vi "Facade.vi"(0 "Data In":T10, 2 "Display State In":T5={"ImageSource"=enum."Camera", "IMAQdx Cam"=refnum, "WorkDir"=path "", "Image Name Prefix"="", "ROI"={"Global Rectangle"=[], "Contours"=[]}, "BG Image"=refnum, "Display Image"=refnum, "Display settings"={"Min. Thresh."=0.0, "X"=0.0, "Y"=0.0, "ShowLineout"=FALSE, "ScaleParts"=10, "ShowLegende"=FALSE, "Target Cross"=FALSE, "Centroid Cross"=FALSE, "Target color"=16777226, "Centroid color"=16711680, "calibr. mm/px"=0.0}, "Mask image"=refnum, "ConfigDir"=path "", "Display ref"=refnum, "Saved ROIs"=[], "Selected ROI"="", "Analyze Objects"=[], "Analysis Params"=variant, "Analysis Results"=variant, "Overlays?"=[], "Ref Palette type"=refnum, "Time in Filename?"=TRUE, "Save Report?"=TRUE, "Appl Params"=variant, "Show ZoomBtn?"=TRUE, "Image file"=path ""} {"ROI"."Contours"."Type" items=["No Selection", "Point", "Line", "Rectangle", "Oval", "Polygon", "Freehand Region", "Annulus", "Unused2", "Unused3", "Broken Line", "Freehand Line", "Rotated Rectangle"]}, 3 "Container State":T9) -> (6 "Data Out":T10, 7 "Display State Out":T5={"ImageSource"=enum."Camera", "IMAQdx Cam"=refnum, "WorkDir"=path "", "Image Name Prefix"="", "ROI"={"Global Rectangle"=[], "Contours"=[]}, "BG Image"=refnum, "Display Image"=refnum, "Display settings"={"Min. Thresh."=0.0, "X"=0.0, "Y"=0.0, "ShowLineout"=FALSE, "ScaleParts"=10, "ShowLegende"=FALSE, "Target Cross"=FALSE, "Centroid Cross"=FALSE, "Target color"=16777226, "Centroid color"=16711680, "calibr. mm/px"=0.0}, "Mask image"=refnum, "ConfigDir"=path "", "Display ref"=refnum, "Saved ROIs"=[], "Selected ROI"="", "Analyze Objects"=[], "Analysis Params"=variant, "Analysis Results"=variant, "Overlays?"=[], "Ref Palette type"=refnum, "Time in Filename?"=TRUE, "Save Report?"=TRUE, "Appl Params"=variant, "Show ZoomBtn?"=TRUE, "Image file"=path ""} {"ROI"."Contours"."Type" items=["No Selection", "Point", "Line", "Rectangle", "Oval", "Polygon", "Freehand Region", "Annulus", "Unused2", "Unused3", "Broken Line", "Freehand Line", "Rotated Rectangle"]}, 8 "Action":T4)   [LabVIEW 2020, in "POLARIS IMAQ Display.xctl"]
uses:
  POLARIS IMAQ Display.xctl
  Data.ctl
  <vilib>/vision/Image Controls.llb/IMAQ Image.ctl
  <vilib>/_xctls/Container State.ctl
  State.ctl
  IMAQdx Cam/IMAQdx Cam.lvclass
  Properties/ImageSource.ctl
  DisplaySettings.ctl
  Named ROI.ctl
  Analyze Classes/Analyze BaseClass/Analyze BaseClass.lvclass
  Palette.ctl
  <vilib>/_xctls/Action.ctl
  <vilib>/_xctls/XControlSupport.lvlib
  Utility/POLARIS Vision utility.lvlib
  <vilib>/vision/NI_Vision_Development_Module.lvlib
  <vilib>/Utility/config.llb/NI_LVConfig.lvlib
panel:
  in  "Zoom Buttons":enum32{"Zoom in", "Zoom out", "Zenter"}(radio)
  in  "Pallete":T1={"Teiler"=1, "Palette Type"=0} {"Teiler" min=1 max=5; "Palette Type" items=["Grayscale", "Binary", "Gradient", "Rainbow", "Temperature", "User Defined"]}
  in  "Report File":path
  in  "ROI Name":string
  out "Display settings":T2={"Min. Thresh."=0.0, "X"=0.0, "Y"=0.0, "ShowLineout"=FALSE, "ScaleParts"=10, "ShowLegende"=FALSE, "Target Cross"=FALSE, "Centroid Cross"=FALSE, "Target color"=16777226, "Centroid color"=16711680, "calibr. mm/px"=0.0}
  out "Centroid":cluster{"X Centroid":sgl, "Y Centroid":sgl} {"Y Centroid" format="%.2f"; "X Centroid" format="%.2f"}
  in  "Sub\nBG":bool
  out "error out":errorcluster
  out "Image":T3(plugin-control)
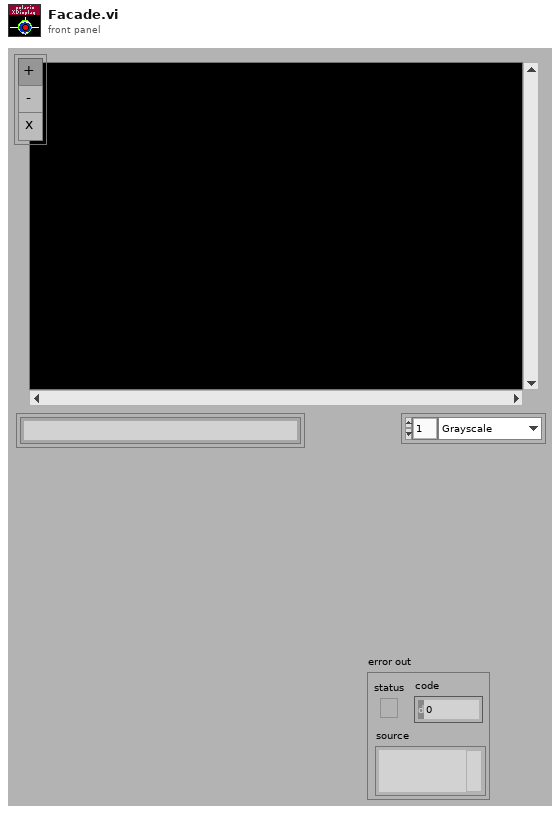
[diagram p1: front panel]
types:
  T1 = typedef "POLARIS IMAQ Display.xctl/Palette.ctl" = cluster{"Teiler":i32, "Palette Type":u32}
  T2 = typedef "POLARIS IMAQ Display.xctl/DisplaySettings.ctl" = cluster{"Min. Thresh.":sgl, "X":dbl, "Y":dbl, "ShowLineout":bool, "ScaleParts":i32, "ShowLegende":bool, "Target Cross":bool, "Centroid Cross":bool, "Target color":u32, "Centroid color":u32, "calibr. mm/px":sgl}
  T3 = typedef "IMAQ Image.ctl" = refnum<image>
  T4 = typedef "XControlSupport.lvlib/Action.ctl" = cluster{"Data Changed?":bool, "State Changed?":bool, "Action Name":string}
  T5 = typedef "POLARIS IMAQ Display.xctl/State.ctl" = cluster{"ImageSource":T6, "IMAQdx Cam":refnum<class "IMAQdx Cam.lvclass">, "WorkDir":path, "Image Name Prefix":string, "ROI":T7, "BG Image":T3, "Display Image":T3, "Display settings":T2, "Mask image":T3, "ConfigDir":path, "Display ref":refnum<vi>, "Saved ROIs":T8[], "Selected ROI":string, "Analyze Objects":refnum<class "Analyze BaseClass.lvclass">[], "Analysis Params":variant, "Analysis Results":variant, "Overlays?":bool[], "Ref Palette type":refnum<vi>, "Time in Filename?":bool, "Save Report?":bool, "Appl Params":variant, "Show ZoomBtn?":bool, "Image file":path}
  T6 = typedef "POLARIS IMAQ Display.xctl/ImageSource.ctl" = enum16{"Camera", "File"}
  T7 = typedef "ROI Descriptor" = cluster{"Global Rectangle":i32[], "Contours":cluster{"ID":enum32{"External", "Internal"}, "Type":u32, "Coordinates":i32[]}[]}
  T8 = typedef "POLARIS IMAQ Display.xctl/Named ROI.ctl" = cluster{"ROI":cluster{"Global Rectangle":i32[], "Contours":cluster{"Contour Type":u32, "ROI Type":u32, "Points":i32[]}[]}, "Name":string}
  T9 = typedef "XControlSupport.lvlib/Container State.ctl" = cluster{"Indicator?":bool, "Run Mode?":bool, " Refnum":refnum<vi>}
  T10 = typedef "POLARIS IMAQ Display.xctl/Data.ctl" = cluster{"Image":T3}
  T11 = typedef "Image Type" = u32
  T12 = cluster{"Global Rectangle":i32[], "Contours":cluster{"Contour Type":u32, "ROI Type":u32, "Points":i32[]}[]}
  T13 = typedef "IMAQdx.ctl" = refnum<k21>
  T14 = typedef "NI_LVConfig.lvlib/Config Data RefNum.ctl" = refnum<k1>
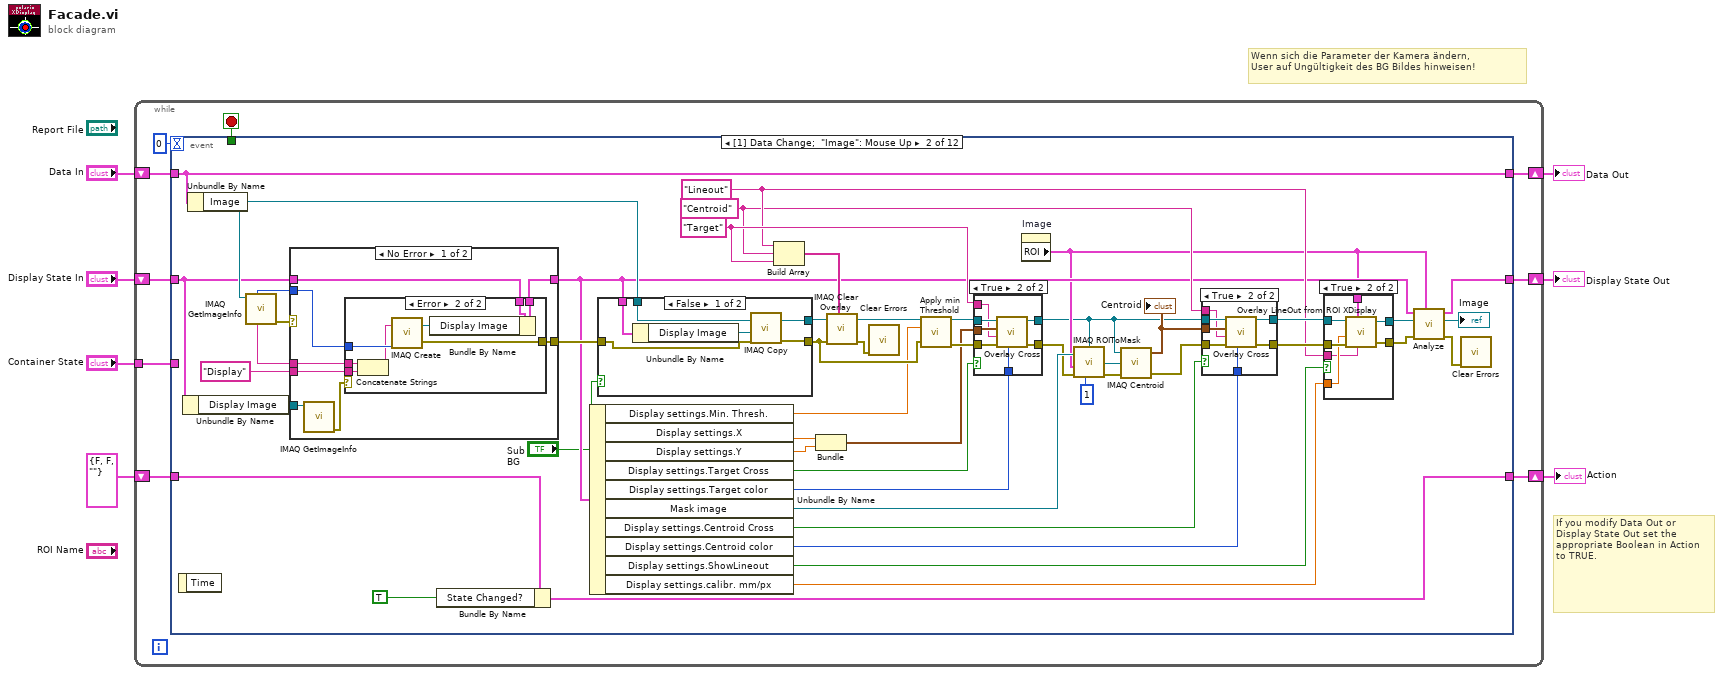
[diagram p0: block diagram]
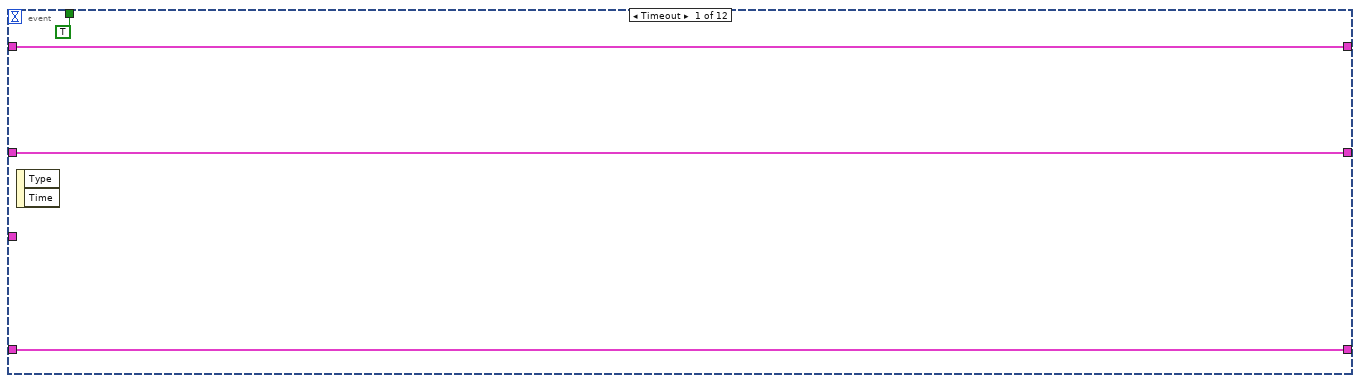
[diagram p2: hidden frame]
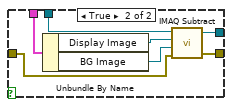
[diagram p8: hidden frame]
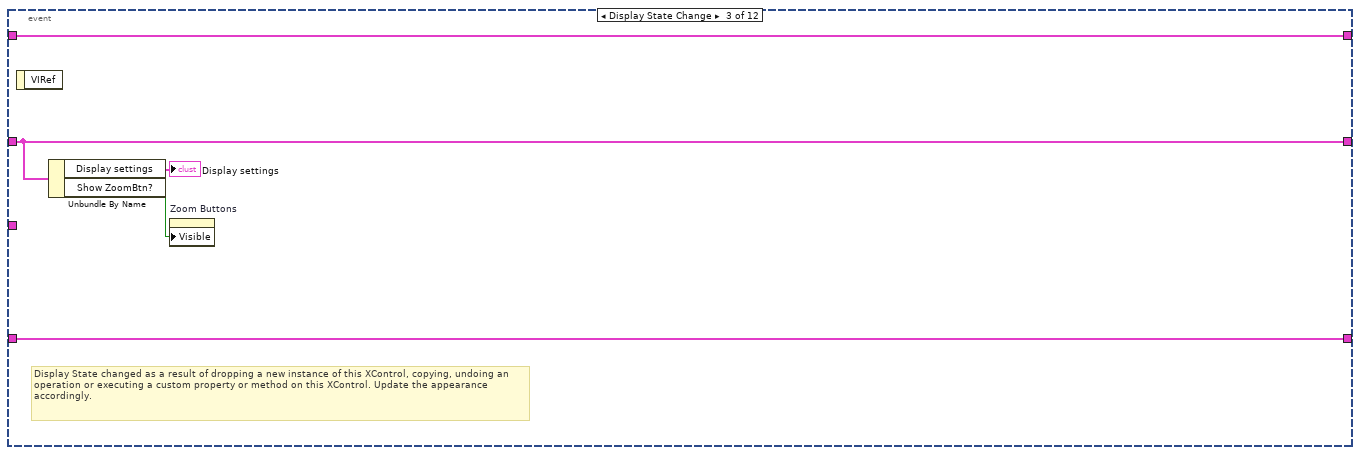
[diagram p9: hidden frame]
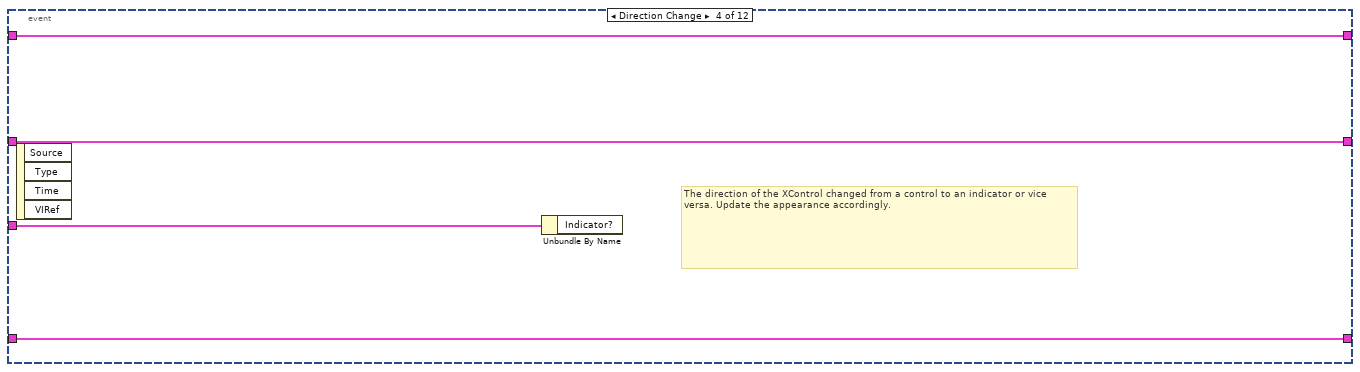
[diagram p10: hidden frame]
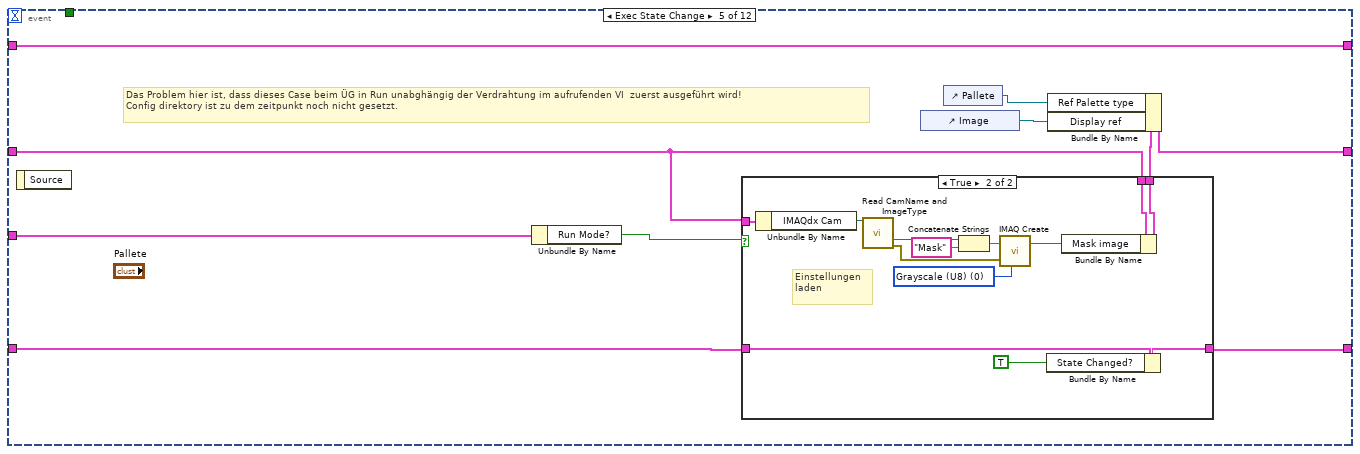
[diagram p11: hidden frame]
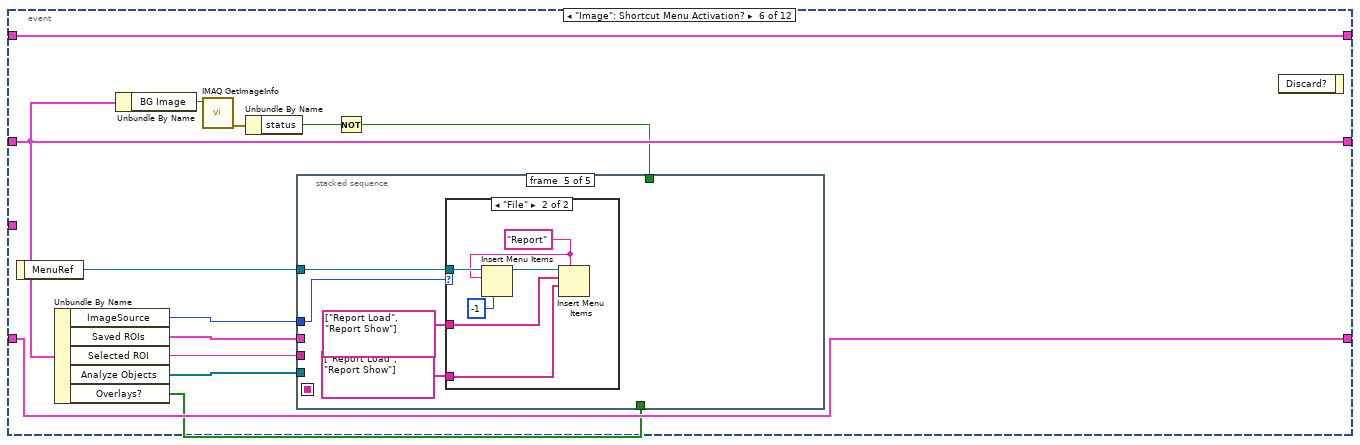
[diagram p13: hidden frame]
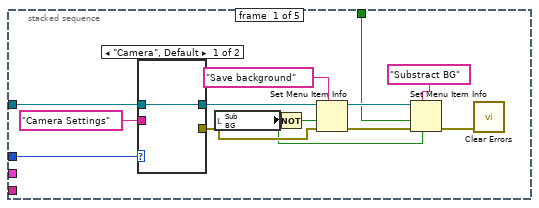
[diagram p14: hidden frame]
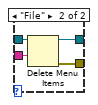
[diagram p15: hidden frame]
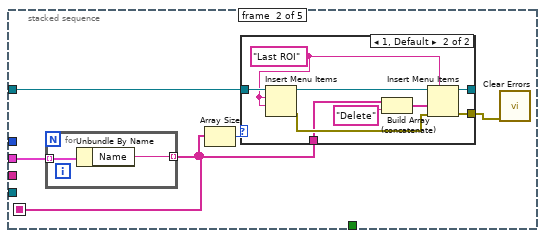
[diagram p16: hidden frame]
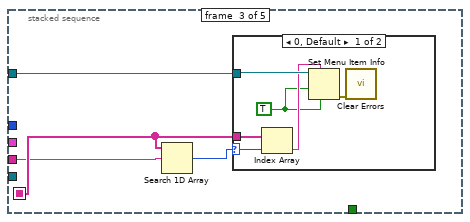
[diagram p18: hidden frame]
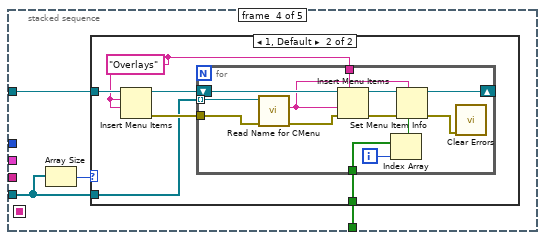
[diagram p20: hidden frame]
diagram:
  # "Wenn sich die Parameter der Kamera ändern,\nUser auf Ungültigkeit des BG Bildes hinweisen!"
  # "If you modify Data Out or\nDisplay State Out set the\nappropriate Boolean in Action\nto TRUE."
  n1 = while {
    shift-right: [w15] -> w4
    shift-left: "Display State In" -> [w16]
    tunnel: "Container State" -> [w12]
    shift-right: [w11] -> w7
    shift-left: "Data In" -> [w8]
    shift-right: [w9] -> w2
    shift-left: T4 {"Data Changed?"=FALSE, "State Changed?"=FALSE, "Action Name"=""} ("Action") -> [w10]
    stop <- w14 stop-if-true
    n2 = event shown="[1] Data Change;  \"Image\": Mouse Up" {
      selector: _ -> [_ _ _ _ _ _ _ _ _ _ _ _]
      dyn-events: _ -> [_ _ _ _ _ _ _ _ _ _ _ _]
      timeout: 0 -> [_ _ _ _ _ _ _ _ _ _ _ _]
      tunnel: w16 -> [w18 w23 w131 w137 w145 w174 w260 w426 w437 w451 w457 w462]
      tunnel: [w18 w32 w131 w137 w141 w174 w258 w425 w431 w442 w457 w462] -> w15
      tunnel: [TRUE _ _ _ _ _ _ _ _ _ _ _] -> w14
      tunnel: w12 -> [_ _ _ w138 w148 _ w255 _ _ _ _ _]
      tunnel: w8 -> [w17 w70 w134 w136 w147 w176 w259 w429 w441 w450 w456 w461]
      tunnel: [w17 w70 w134 w136 w147 w176 w259 w429 w441 w450 w456 w461] -> w11
      tunnel: [w19 w46 w132 w135 w142 w175 w256 w416 w434 w448 w455 w460] -> w9
      tunnel: w10 -> [w19 w47 w132 w135 w143 w175 w257 w428 w440 w449 w455 w460]
      event Timeout {
        n3 = event-data() -> ()  [unwired: 1 in, 2 out]
      }
      event Data Change; "Image": Mouse Up {
        w38 = "Lineout" ("Group")
        w39 = "Target"
        w37 = "Centroid"
        n4 = event-data() -> ()  [unwired: 1 in, 1 out]
        n5 = Unbundle By Name(w23) -> ("Display Image"=w22:T3)
        n6 = Unbundle By Name(w70) -> ("Image"=w44:T3)
        n7 = call "IMAQ GetImageInfo"("Image"=w44) -> ("error out"=w41:errorcluster, "Image Name"=w43:string, "Image Type"=w42:T11)  [unwired: 3 in, 5 out]
        n8 = case shown="No Error" w41 {
          selector: w41 -> [_ w88]
          tunnel: w23 -> [w78 w89]
          tunnel: [w77 w89] -> w33
          tunnel: [w76 w88] -> w45
          tunnel: w43 -> [w75 _]
          tunnel: w42 -> [w74 _]
          tunnel: "Display" ("string") -> [w73 _]
          tunnel: w22 -> [w72 _]
          frame No Error {
            n9 = call "IMAQ GetImageInfo"("Image"=w72) -> ("error out"=w71:errorcluster)  [unwired: 3 in, 7 out]
            n10 = case shown="Error" w71 {
              tunnel: w78 -> [w79 w87]
              tunnel: [w79 w86] -> w77
              tunnel: [_ w85] -> w76
              tunnel: w75 -> [_ w84]
              tunnel: w74 -> [_ w83]
              tunnel: w73 -> [_ w80]
              frame No Error {
              }
              frame Error {
                n11 = Concatenate Strings(w84, w80) -> (w82:string)
                n12 = call "IMAQ Create"("Image Name"=w82, "Image Type"=w83) -> ("New Image"=w81:T3, "error out"=w85:errorcluster)  [unwired: 3 in]
                n13 = Bundle By Name(cluster=w87, "Display Image"=w81) -> (w86:T5)
              }
            }
          }
          frame Error {
          }
        }
        n14 = Bundle By Name(cluster=w47, "State Changed?"=TRUE) -> (w46:T4)
        n15 = Unbundle By Name(w33) -> ("Display settings.Min. Thresh."=w24:sgl, "Display settings.X"=w67:dbl, "Display settings.Y"=w66:dbl, "Display settings.Target Cross"=w65:bool, "Display settings.Target color"=w63:u32, "Mask image"=w59:T3, "Display settings.Centroid Cross"=w58:bool, "Display settings.Centroid color"=w55:u32, "Display settings.ShowLineout"=w51:bool, "Display settings.calibr. mm/px"=w50:sgl)
        n16 = case shown="False" "Sub\nBG" {
          tunnel: w33 -> [w122 w129]
          tunnel: w44 -> [w121 w126]
          tunnel: [w119 w127] -> w49
          tunnel: [w118 w124] -> w35
          tunnel: w45 -> [w117 w123]
          frame False {
            n17 = Unbundle By Name(w122) -> ("Display Image"=w120:T3)
            n18 = call "IMAQ Copy"("error in (no error)"=w117, "Image Dst"=w120, "Image Src"=w121) -> ("error out"=w118:errorcluster, "Image Dst Out"=w119:T3)  [unwired: 3 in]
          }
          frame True {
            n19 = Unbundle By Name(w129) -> ("Display Image"=w125:T3, "BG Image"=w128:T3)
            n20 = call "IMAQ Subtract"("Image Src A"=w126, "Image Dst"=w125, "Image Src B"=w128, "error in (no error)"=w123) -> ("Image Dst Out"=w127:T3, "error out"=w124:errorcluster)  [unwired: 3 in]
          }
        }
        n21 = Build Array(w38, w37, w39) -> (w36:string[])
        n22 = Bundle("X"=w67, "Y"=w66) -> (w64:cluster{"X":dbl, "Y":dbl})  [unwired: 1 in]
        n23 = call "IMAQ Clear Overlay"("Groups"=w36, "error in (no error)"=w35, "Image"=w49) -> ("error out"=w34:errorcluster, "Image Out"=w48:T3)  [unwired: 7 in]
        n24 = call <vilib>:"Clear Errors.vi"("error in (no error)"=w34) -> ()  [unwired: 5 in, 2 out]
        n25 = call "Apply min Threshold.vi"("error in"=w35, "Min. Thresh."=w24, "Image In"=w48) -> ("error out"=w68:errorcluster, "Image Out"=w69:T3)  [unwired: 7 in]
        n26 = case shown="True" w65 {
          tunnel: w69 -> [w109 w116]
          tunnel: [w109 w115] -> w21
          tunnel: w68 -> [w108 w114]
          tunnel: w64 -> [_ w113]
          tunnel: w63 -> [_ w112]
          tunnel: [w108 w111] -> w57
          tunnel: w39 -> [_ w110]
          frame False {
          }
          frame True {
            n27 = call "Overlay Cross.vi"("Color"=w112, "error in (no error)"=w114, "Overlay Group"=w110, "point"=w113, "Image In"=w116) -> ("error out"=w111:errorcluster, "Image Out"=w115:T3)  [unwired: 4 in]
          }
        }
        n28 = property on="Image" class="ImageControl"() -> ("ROI"=w27:T12)  [unwired: 2 in, 2 out]
        n29 = call "IMAQ ROIToMask"("error in (no error)"=w57, "ROI Descriptor"=w27, "Filling Value (255)"=1, "Image"=w59, "Image Model"=w21) -> ("error out"=w62:errorcluster, "Image Out"=w61:T3)  [unwired: 1 in, 1 out]
        n30 = call "IMAQ Centroid"("error in (no error)"=w62, "Image Mask"=w61, "Image"=w21) -> ("error out"=w56:errorcluster, "Centroid"=w54:cluster{"X Centroid":sgl, "Y Centroid":sgl})  [unwired: 1 in]
        "Centroid" <- w54
        n31 = case shown="True" w58 {
          tunnel: w21 -> [w100 w107]
          tunnel: [w100 w106] -> w53
          tunnel: w56 -> [w99 w105]
          tunnel: w54 -> [_ w104]
          tunnel: w55 -> [_ w103]
          tunnel: [w99 w102] -> w52
          tunnel: w37 -> [_ w101]
          frame False {
          }
          frame True {
            n32 = call "Overlay Cross.vi"("Color"=w103, "error in (no error)"=w105, "Overlay Group"=w101, "point"=w104, "Image In"=w107) -> ("error out"=w102:errorcluster, "Image Out"=w106:T3)  [unwired: 4 in]
          }
        }
        n33 = case shown="True" w51 {
          tunnel: w53 -> [w91 w98]
          tunnel: w52 -> [w90 w97]
          tunnel: w27 -> [_ w96]
          tunnel: [w91 w95] -> w31
          tunnel: [w90 w94] -> w29
          tunnel: w50 -> [_ w93]
          tunnel: w38 -> [_ w92]
          frame False {
          }
          frame True {
            n34 = call "Overlay LineOut from ROI XDisplay.vi"("Image In"=w98, "ROI"=w96, "Calbration"=w93, "Group"=w92, "error in"=w97) -> ("Image Out"=w95:T3, "error out"=w94:errorcluster)  [unwired: 1 in, 1 out]
          }
        }
        n35 = call "Analyze.vi"("ROI"=w27, "error in"=w29, "Image in"=w31, "State in"=w33) -> ("error out"=w28:errorcluster, "Image out"=→"Image":T3, "State out"=w32:T5)  [unwired: 5 in]
        n36 = call <vilib>:"Clear Errors.vi"("error in (no error)"=w28) -> ()  [unwired: 5 in, 2 out]
      }
      event Display State Change {
        # "Display State changed as a result of dropping a new instance of this XControl, copying, undoing an operation or executing a custom property or method on this XControl. Update the appearance accordingly."
        n37 = event-data() -> ()  [unwired: 1 in, 1 out]
        n38 = Unbundle By Name(w131) -> ("Display settings"=→"Display settings":T2, "Show ZoomBtn?"=w130:bool)
        n39 = property on="Zoom Buttons" class="RadioBtnsControl (strict)"("Visible"=w130) -> ()  [unwired: 2 in, 2 out]
      }
      event Direction Change {
        # "The direction of the XControl changed from a control to an indicator or vice versa. Update the appearance accordingly."
        n40 = event-data() -> ()  [unwired: 1 in, 4 out]
        n41 = Unbundle By Name(w138) -> ()  [unwired: 1 out]
      }
      event Exec State Change {
        # "Das Problem hier ist, dass dieses Case beim ÜG in Run unabghängig der Verdrahtung im aufrufenden VI  zuerst ausgeführt wird!\nConfig direktory ist zu dem zeitpunkt noch nicht gesetzt."
        n42 = event-data() -> ()  [unwired: 1 in, 1 out]
        n43 = Unbundle By Name(w148) -> ("Run Mode?"=w146:bool)
        n44 = case shown="True" w146 {
          tunnel: w145 -> [_ w163]
          tunnel: w145 -> [w150 w157]
          tunnel: [w150 w152] -> w144
          tunnel: w143 -> [w149 w154]
          tunnel: [w149 w153] -> w142
          frame False {
          }
          frame True {
            w155 = T11 0 items=["Grayscale (U8)", "Grayscale (I16)", "Grayscale (SGL)", "Complex (CSG)", "RGB (U32)", "HSL (U32)", "RGB (U64)", "Grayscale (U16)"] ("Image Type")
            # "Einstellungen\nladen"
            n45 = Unbundle By Name(w163) -> ("IMAQdx Cam"=w162:refnum<class "IMAQdx Cam.lvclass">)
            n46 = call-dynamic "Read CamName and ImageType.vi"("IMAQdx Cam in"=w162) -> ("error out"=w158:errorcluster, "Camera"=w161:T13)  [unwired: 7 in, 2 out]
            n47 = Concatenate Strings(w161, "Mask" ("string")) -> (w159:string)
            n48 = call "IMAQ Create"("Image Name"=w159, "Image Type"=w155, "error in (no error)"=w158) -> ("New Image"=w156:T3)  [unwired: 2 in, 1 out]
            n49 = Bundle By Name(cluster=w154, "State Changed?"=TRUE ("Data Changed?")) -> (w153:T4)
            n50 = Bundle By Name(cluster=w157, "Mask image"=w156) -> (w152:T5)
          }
        }
        n51 = control-ref of="Image"() -> (w140:refnum<vi>)
        n52 = control-ref of="Pallete"() -> (w139:refnum<vi>)
        n53 = Bundle By Name(cluster=w144, "Ref Palette type"=w139, "Display ref"=w140) -> (w141:T5)
      }
      event "Image": Shortcut Menu Activation? {
        n54 = event-data() -> ("MenuRef"=w170:refnum<k9>)  [unwired: 1 in]
        n55 = Unbundle By Name(w174) -> ("ImageSource"=w164:T6, "Saved ROIs"=w169:T8[], "Selected ROI"=w168:string, "Analyze Objects"=w166:refnum<class "Analyze BaseClass.lvclass">[], "Overlays?"=w165:bool[])
        n56 = Unbundle By Name(w174) -> ("BG Image"=w173:T3)
        n57 = call "IMAQ GetImageInfo"("Image"=w173) -> ("error out"=w172:errorcluster)  [unwired: 3 in, 7 out]
        n58 = Unbundle By Name(w172) -> ("status"=w171:bool)
        n59 = Not(x=w171) -> (.not. x?=w167:bool)
        n60 = stacked-sequence {
          seq-local: [_ w197 _ _ _] -> [_ _ w214 _ _]
          tunnel: w170 -> [w182 w199 w215 w224 w248]
          tunnel: w169 -> [_ w198 _ _ _]
          tunnel: w168 -> [_ _ w213 _ _]
          tunnel: w167 -> [w178 _ _ _ _]
          tunnel: w166 -> [_ _ _ w222 _]
          tunnel: w165 -> [_ _ _ w223 _]
          tunnel: w164 -> [w180 _ _ _ w247]
          frame #0 {
            n61 = case shown="\"Camera\", Default" w180 {
              tunnel: w182 -> [w190 w194]
              tunnel: [w190 w193] -> w186
              tunnel: [_ w192] -> w183
              tunnel: "Camera Settings" ("menu tag") -> [_ w191]
              frame "Camera", Default {
              }
              frame "File" {
                n62 = Delete Menu Items(7:w191, 9:w194) -> (0:w192:errorcluster, 3:w193:refnum<k9>)  [unwired: 2 in]
              }
            }
            n63 = local read "Sub\nBG"() -> (w177:bool)
            n64 = Not(x=w177) -> (.not. x?=w185:bool)
            n65 = Set Menu Item Info(7:"Save background" ("item tag"), 8:w183, 9:w185, 11:w186) -> (0:w188:errorcluster, 3:w187:refnum<k9>)  [unwired: 3 in]
            n66 = Set Menu Item Info(6:w177, 7:"Substract BG" ("item tag"), 8:w188, 9:w178, 11:w187) -> (0:w179:errorcluster)  [unwired: 2 in, 1 out]
            n67 = call <vilib>:"Clear Errors.vi"("error in (no error)"=w179) -> ()  [unwired: 5 in, 2 out]
          }
          frame #1 {
            n68 = for {
              tunnel: w198 -> [w211] mode=indexing
              tunnel: [w210] -> w197 mode=indexing
              n69 = Unbundle By Name(w211) -> ("Name"=w210:string)
            }
            n70 = Array Size(array=w197) -> (size(s)=w196:i32)
            n71 = case shown="1, Default" w196 {
              tunnel: w199 -> [w200 w208]
              tunnel: w197 -> [_ w205]
              tunnel: [w200 w204] -> _
              tunnel: [_ w203] -> w195
              frame 0 {
              }
              frame 1, Default {
                w201 = "Last ROI" ("menu tag")
                n72 = Insert Menu Items(7:w201, 8:w201, 9:w208) -> (0:w209:errorcluster, 3:w207:refnum<k9>)  [unwired: 3 in, 1 out]
                n73 = Build Array (concatenate)(w205, "Delete" ("item names")) -> (w202:string[])
                n74 = Insert Menu Items(5:w201, 6:w209, 7:w202, 9:w207) -> (0:w203:errorcluster, 3:w204:refnum<k9>)  [unwired: 2 in, 1 out]
              }
            }
            n75 = call <vilib>:"Clear Errors.vi"("error in (no error)"=w195) -> ()  [unwired: 5 in, 2 out]
          }
          frame #2 {
            n76 = Search 1D Array(1D array=w214, element=w213) -> (index of element=w212:i32)  [unwired: 1 in]
            n77 = case shown="0, Default" w212 {
              selector: w212 -> [w220 _]
              tunnel: w214 -> [w219 _]
              tunnel: w215 -> [w221 _]
              frame 0, Default {
                w217 = TRUE ("checked")
                n78 = Index Array(array=w219, index=w220) -> (element=w218:string)
                n79 = Set Menu Item Info(6:w217, 7:w218, 9:w217, 11:w221) -> (0:w216:errorcluster)  [unwired: 3 in, 1 out]
                n80 = call <vilib>:"Clear Errors.vi"("error in (no error)"=w216) -> ()  [unwired: 5 in, 2 out]
              }
              frame -1 {
              }
            }
          }
          frame #3 {
            n81 = Array Size(array=w222) -> (size(s)=w225:i32)
            n82 = case shown="1, Default" w225 {
              tunnel: w224 -> [_ w231]
              tunnel: w222 -> [_ w228]
              tunnel: w223 -> [_ w227]
              frame 0 {
              }
              frame 1, Default {
                w226 = "Overlays" ("menu tag")
                n83 = Insert Menu Items(7:w226, 8:w226, 9:w231) -> (0:w229:errorcluster, 3:w230:refnum<k9>)  [unwired: 3 in, 1 out]
                n84 = for {
                  tunnel: w229 -> [w237]
                  tunnel: w228 -> [w238] mode=indexing
                  tunnel: w226 -> [w243]
                  tunnel: w227 -> [w233]
                  shift-right: [w240] -> _
                  shift-left: w230 -> [w244]
                  i -> [w232]
                  n85 = call-dynamic "Read Name for CMenu.vi"("error in (no error)"=w237, "Analyze BaseClass in"=w238) -> ("error out"=w236:errorcluster, "Name for Context menu"=w235:string)  [unwired: 7 in, 1 out]
                  n86 = Insert Menu Items(5:w243, 6:w236, 7:w235, 9:w244) -> (0:w241:errorcluster, 3:w242:refnum<k9>)  [unwired: 2 in, 1 out]
                  n87 = Index Array(array=w233, index=w232) -> (element=w234:bool)
                  n88 = Set Menu Item Info(6:w234, 7:w235, 8:w241, 11:w242) -> (0:w239:errorcluster, 3:w240:refnum<k9>)  [unwired: 3 in]
                  n89 = call <vilib>:"Clear Errors.vi"("error in (no error)"=w239) -> ()  [unwired: 5 in, 2 out]
                }
              }
            }
          }
          frame #4 {
            n90 = case shown="\"File\"" w247 {
              tunnel: w248 -> [_ w253]
              tunnel: string[] ["Report Load", "Report Show"] ("item names") -> [_ w254]
              tunnel: string[] ["Report Load", "Report Show"] ("item names") -> [_ w249]
              frame "Camera", Default {
              }
              frame "File" {
                w251 = "Report" ("menu tag")
                n91 = Insert Menu Items(4:-1, 8:w251, 9:w253) -> (3:w252:refnum<k9>)  [unwired: 3 in, 2 out]
                n92 = Insert Menu Items(5:w251, 7:w249, 8:w254, 9:w252) -> ()  [unwired: 2 in, 3 out]
              }
            }
          }
        }
        n93 = event-data() -> ()  [unwired: 2 in, 1 out]
      }
      event "Image": Shortcut Menu Selection (User) {
        n94 = event-data() -> ("ItemTag"=w261:string)  [unwired: 1 in]
        n95 = case shown="\"Report Load\"" w261 {
          selector: w261 -> [_ _ _ _ _ _ _ _ _ w338 _ _ _]
          tunnel: w260 -> [w266 w274 w293 w308 w321 w326 w330 w334 w337 w340 w385 w405 w410]
          tunnel: w259 -> [_ _ w298 _ _ _ _ _ _ _ _ _ _]
          tunnel: [w266 w274 w289 w299 w321 w325 w330 w334 w337 w339 w384 w405 w409] -> w258
          tunnel: w257 -> [w262 w280 w283 w309 w322 w327 w329 w333 w336 w343 w386 w406 w414]
          tunnel: [w262 w280 w282 w302 w322 w327 w329 w333 w336 w342 w383 w406 w408] -> w256
          tunnel: w255 -> [_ _ _ _ _ w324 _ _ _ _ _ _ w412]
          frame "Camera Settings" {
            n96 = Unbundle By Name(w266) -> ("IMAQdx Cam"=w265:refnum<class "IMAQdx Cam.lvclass">)
            n97 = call-dynamic "Open camera settings.vi"("IMAQdx Cam in"=w265) -> ("error out"=w264:errorcluster)  [unwired: 9 in, 1 out]
            "error out" <- w264
            n98 = case shown="True" FALSE {
              tunnel: w264 -> [_ w267]
              frame False {
              }
              frame True {
                n99 = Open VI Reference(vi path=path "New BG Msg.vi", error in (no error)=w267) -> (vi reference=w271:refnum<vi>, error out=w270:errorcluster)  [unwired: 4 in]
                n100 = invoke class="VI" method="FP.Open"(reference=w271, error in=w270, "Activate"=TRUE ("Wait Until Done")) -> (error out=w268:errorcluster)  [unwired: 2 in, 4 out]
                n101 = call <vilib>:"Clear Errors.vi"("error in (no error)"=w268) -> ()  [unwired: 5 in, 2 out]
              }
            }
          }
          frame "Load ROI from File" {
            n102 = Unbundle By Name(w274) -> ("IMAQdx Cam"=w279:refnum<class "IMAQdx Cam.lvclass">)
            n103 = call-dynamic "Read CamName and ImageType.vi"("IMAQdx Cam in"=w279) -> ("error out"=w276:errorcluster, "Camera"=w275:T13)  [unwired: 7 in, 2 out]
            n104 = control-ref of="Report File"() -> (w273:refnum<vi>)
            n105 = call "Open Dialog VI.vi"("error in"=w276, "Windows title"=w275, "ref for signalling"=w273, "vi path"=path "Load Settings from Report.vi") -> ("error out"=w278:errorcluster)  [unwired: 7 in]
            n106 = call <vilib>:"Clear Errors.vi"("error in (no error)"=w278) -> ()  [unwired: 5 in, 2 out]
          }
          frame "Save background" {
            n107 = Unbundle By Name(w298) -> ("Image"=w291:T3)
            n108 = call "IMAQ GetImageInfo"("Image"=w291) -> ("error out"=w288:errorcluster, "Image Name"=w296:string, "Image Type"=w297:T11)  [unwired: 3 in, 5 out]
            n109 = Concatenate Strings(w296, "_BG" ("string")) -> (w295:string)
            n110 = call "IMAQ Create"("Image Name"=w295, "Image Type"=w297, "error in (no error)"=w288) -> ("New Image"=w292:T3, "error out"=w287:errorcluster)  [unwired: 2 in]
            n111 = Bundle By Name(cluster=w283, "State Changed?"=TRUE) -> (w282:T4)
            n112 = call "IMAQ Copy"("error in (no error)"=w287, "Image Dst"=w292, "Image Src"=w291) -> ("error out"=w286:errorcluster, "Image Dst Out"=w290:T3)  [unwired: 3 in]
            n113 = Unbundle By Name(w286) -> ("status"=w285:bool)
            n114 = Not(x=w285) -> (.not. x?=w284:bool)
            n115 = local write "Sub\nBG"(w284) -> ()
            n116 = Bundle By Name(cluster=w293, "BG Image"=w290) -> (w289:T5)
          }
          frame "Delete" {
            # "Delete named ROI"
            n117 = Unbundle By Name(w308) -> ("Saved ROIs"=w305:T8[], "Selected ROI"=w307:string)
            n118 = for {
              tunnel: w305 -> [w311] mode=indexing
              tunnel: [w310] -> w306 mode=indexing
              n119 = Unbundle By Name(w311) -> ("Name"=w310:string)
            }
            n120 = Bundle By Name(cluster=w309, "State Changed?"=TRUE) -> (w302:T4)
            n121 = Search 1D Array(1D array=w306, element=w307) -> (index of element=w304:i32)  [unwired: 1 in]
            n122 = Delete From Array(array=w305, index=w304) -> (array with subset deleted=w303:T8[])  [unwired: 1 in, 1 out]
            n123 = Bundle By Name(cluster=w308, "Saved ROIs"=w303) -> (w299:T5)
            n124 = call "Write Display Settings 2 File.vi"("State"=w299) -> ("error out"=w300:errorcluster)  [unwired: 9 in, 1 out]
            n125 = call <vilib>:"Clear Errors.vi"("error in (no error)"=w300) -> ()  [unwired: 5 in, 2 out]
          }
          frame "Display settings" {
            n126 = Unbundle By Name(w321) -> ("Display settings"=w314:T2, "IMAQdx Cam"=w320:refnum<class "IMAQdx Cam.lvclass">)
            n127 = control-ref of="Display settings"() -> (w315:refnum<vi>)
            n128 = property class="Clust (strict)"(reference=w315, "Value"=w314) -> (reference out=w312:refnum<vi>, error out=w313:errorcluster)  [unwired: 1 in]
            n129 = call-dynamic "Read CamName and ImageType.vi"("error in (no error)"=w313, "IMAQdx Cam in"=w320) -> ("error out"=w317:errorcluster, "Camera"=w316:T13)  [unwired: 6 in, 2 out]
            n130 = call "Open Dialog VI.vi"("error in"=w317, "Windows title"=w316, "ref for signalling"=w312, "vi path"=path "Display Settings.vi") -> ("error out"=w319:errorcluster)  [unwired: 7 in]
            n131 = call <vilib>:"Clear Errors.vi"("error in (no error)"=w319) -> ()  [unwired: 5 in, 2 out]
          }
          frame "Save Image" {
            n132 = call "Save Image.vi"("Display State In"=w326, "Container State"=w324) -> ("Display State Out"=w325:T5, "error out"=w323:errorcluster)  [unwired: 12 in]
            n133 = call <vilib>:"Clear Errors.vi"("error in (no error)"=w323) -> ()  [unwired: 5 in, 2 out]
          }
          frame "Clear ROI" {
            n134 = invoke on="Image" class="ImageControl" method="Clear ROI"() -> (error out=w328:errorcluster)  [unwired: 3 in, 2 out]
            n135 = call <vilib>:"Clear Errors.vi"("error in (no error)"=w328) -> ()  [unwired: 5 in, 2 out]
          }
          frame "Substract BG" {
            n136 = local read "Sub\nBG"() -> (w332:bool)
            n137 = Not(x=w332) -> (.not. x?=w331:bool)
            n138 = local write "Sub\nBG"(w331) -> ()
          }
          frame "Show ROI Tools" {
            n139 = call "IMAQ WindToolsShow"() -> ("error out"=w335:errorcluster)  [unwired: 5 in, 1 out]
            n140 = call <vilib>:"Clear Errors.vi"("error in (no error)"=w335) -> ()  [unwired: 5 in, 2 out]
          }
          frame "Last ROI", Default {
            n141 = Unbundle By Name(w340) -> ("Saved ROIs"=w341:T8[])
            n142 = for {
              tunnel: w341 -> [w381] mode=indexing
              tunnel: w338 -> [w379]
              tunnel: [w378] -> w345
              tunnel: [w377] -> w344
              i -> [w377]
              stop <- w378 stop-if-true
              n143 = Unbundle By Name(w381) -> ("Name"=w380:string)
              n144 = Equal?(x=w380, y=w379) -> (x = y?=w378:bool)
            }
            n145 = case shown="False" w345 {
              tunnel: w341 -> [_ w373]
              tunnel: w344 -> [_ w374]
              tunnel: w343 -> [w354 w371]
              tunnel: [w347 w370] -> w342
              tunnel: w340 -> [w353 w368]
              tunnel: [w349 w367] -> w339
              tunnel: w338 -> [w351 _]
              frame False {
                n146 = Unbundle By Name(w353) -> ("Overlays?"=w350:bool[], "Analyze Objects"=w352:refnum<class "Analyze BaseClass.lvclass">[])
                n147 = for {
                  tunnel: w352 -> [w364] mode=indexing
                  tunnel: w351 -> [w362]
                  tunnel: w350 -> [w360]
                  tunnel: [w358] -> w348 mode=indexing
                  i -> [w355]
                  n148 = call-dynamic "Read Name for CMenu.vi"("Analyze BaseClass in"=w364) -> ("error out"=w357:errorcluster, "Name for Context menu"=w363:string)  [unwired: 8 in, 1 out]
                  n149 = Index Array(array=w360, index=w355) -> (element=w356:bool)
                  n150 = Equal?(x=w363, y=w362) -> (x = y?=w361:bool)
                  n151 = Not(x=w356) -> (.not. x?=w359:bool)
                  n152 = Select(t=w359, s=w361, f=w356) -> (s? t:f=w358:bool)
                  n153 = call <vilib>:"Clear Errors.vi"("error in (no error)"=w357) -> ()  [unwired: 5 in, 2 out]
                }
                n154 = Bundle By Name(cluster=w354, "State Changed?"=TRUE) -> (w347:T4)
                n155 = Bundle By Name(cluster=w353, "Overlays?"=w348) -> (w349:T5)
              }
              frame True {
                w365 = TRUE ("Data Changed?")
                n156 = Index Array(array=w373, index=w374) -> (element=w372:T8)
                n157 = Unbundle By Name(w372) -> ("Name"=w366:string, "ROI"=w375:T12)
                n158 = Bundle By Name(cluster=w368, "Selected ROI"=w366) -> (w367:T5)
                n159 = Bundle By Name(cluster=w371, "Data Changed?"=w365, "Action Name"="ROI", "State Changed?"=w365) -> (w370:T4)
                n160 = property on="Image" class="ImageControl"("ROI"=w375) -> (error out=w376:errorcluster)  [unwired: 2 in, 1 out]
                n161 = call <vilib>:"Clear Errors.vi"("error in (no error)"=w376) -> ()  [unwired: 5 in, 2 out]
              }
            }
          }
          frame "Save ROI" {
            n162 = flat-sequence {
              tunnel: w385 -> [w389]
              tunnel: [w387] -> w384
              frame #0 {
                n163 = property on="Image" class="ImageControl"() -> ("ROI"=w391:T12)  [unwired: 2 in, 2 out]
                n164 = Unbundle By Name(w389) -> ("Saved ROIs"=w390:T8[])
                n165 = Bundle By Name(cluster=T8 {"ROI"={"Global Rectangle"=[], "Contours"=[]}, "Name"=""} ("Named ROI"), "ROI"=w391) -> (w392:T8)
                n166 = Build Array (concatenate)(w392, w390) -> (w388:T8[])
                n167 = Bundle By Name(cluster=w389, "Saved ROIs"=w388) -> (w387:T5)
              }
              frame #1 {
                n168 = control-ref of="ROI Name"() -> (w396:refnum<vi>)
                n169 = call "Open Dialog VI.vi"("ref for signalling"=w396, "vi path"=path "Enter ROI Name.vi") -> ("error out"=w394:errorcluster)  [unwired: 9 in]
                n170 = call <vilib>:"Clear Errors.vi"("error in (no error)"=w394) -> ()  [unwired: 5 in, 2 out]
              }
            }
            n171 = Bundle By Name(cluster=w386, "State Changed?"=TRUE) -> (w383:T4)
          }
          frame "Report Show" {
            n172 = Unbundle By Name(w405) -> ("Image file"=w404:path)
            n173 = call <vilib>:"Get File Extension.vi"("file"=w404) -> ("filename without extension"=w400:string)  [unwired: 6 in, 4 out]
            n174 = Strip Path(path=w404) -> (stripped path=w399:path)  [unwired: 1 out]
            n175 = Concatenate Strings("notepad.exe  " ("command line"), w400, ".data" ("string")) -> (w398:string)
            n176 = call <vilib>:"System Exec.vi"("wait until completion? (T)"=FALSE, "working directory"=w399, "command line"=w398) -> ("error out"=w401:errorcluster)  [unwired: 5 in, 3 out]
            n177 = call <vilib>:"Clear Errors.vi"("error in (no error)"=w401) -> ()  [unwired: 5 in, 2 out]
          }
          frame "Report Load" {
            n178 = Unbundle By Name(w410) -> ("Image file"=w411:path)
            n179 = Bundle By Name(cluster=w414, "State Changed?"=TRUE) -> (w408:T4)
            n180 = call "Read Report File.vi"("Display State In"=w410, "Path"=w411, "Container State"=w412) -> ("Display State Out"=w409:T5, "error out"=w413:errorcluster)  [unwired: 11 in]
            n181 = call <vilib>:"Clear Errors.vi"("error in (no error)"=w413) -> ()  [unwired: 5 in, 2 out]
          }
        }
      }
      event "Report File": Value Change {
        n182 = event-data() -> ("NewVal"=w427:path)  [unwired: 1 in]
        n183 = call <vilib>:"Open Config Data.vi"("configuration file path"=w427) -> ("error out"=w422:errorcluster, "refnum"=w423:T14)  [unwired: 8 in, 1 out]
        n184 = call "ROI from INI Section.vi"("error in (no error)"=w422, "refnum in"=w423) -> ("error out"=w420:errorcluster, "ROI"=w417:T7, "refnum out"=w421:T14)  [unwired: 7 in]
        n185 = property on="Image" class="ImageControl"(error in=w420, "ROI"=w417) -> (error out=w419:errorcluster)  [unwired: 1 in, 1 out]
        n186 = Bundle By Name(cluster=w426, "ROI"=w417) -> (w425:T5)
        n187 = Bundle By Name(cluster=w428, "State Changed?"=TRUE) -> (w416:T4)
        n188 = call <vilib>:"Close Config Data.vi"("error in (no error)"=w419, "write file if changed (T)"=FALSE, "refnum"=w421) -> ("error out"=w418:errorcluster)  [unwired: 7 in, 1 out]
        n189 = call <vilib>:"Clear Errors.vi"("error in (no error)"=w418) -> ()  [unwired: 5 in, 2 out]
      }
      event "ROI Name": Value Change {
        n190 = event-data() -> ("NewVal"=w432:string)  [unwired: 1 in]
        n191 = Unbundle By Name(w437) -> ("Saved ROIs"=w436:T8[])
        n192 = Index Array(array=w436) -> (element=w439:T8)  [unwired: 1 in]
        n193 = Bundle By Name(cluster=w439, "Name"=w432) -> (w438:T8)
        n194 = Bundle By Name(cluster=w440, "State Changed?"=TRUE) -> (w434:T4)
        n195 = Replace Array Subset(array=w436, new element=w438) -> (w435:T8[])  [unwired: 1 in]
        n196 = Bundle By Name(cluster=w437, "Saved ROIs"=w435, "Selected ROI"=w432) -> (w431:T5)
        n197 = call "Write Display Settings 2 File.vi"("State"=w431) -> ("error out"=w430:errorcluster)  [unwired: 9 in, 1 out]
        n198 = call <vilib>:"Clear Errors.vi"("error in (no error)"=w430) -> ()  [unwired: 5 in, 2 out]
      }
      event Value Change {
        n199 = event-data() -> ("NewVal"=w444:T2)  [unwired: 1 in]
        n200 = Bundle By Name(cluster=w449, "Data Changed?"=TRUE, "State Changed?"=TRUE, "Action Name"="Display Settings") -> (w448:T4)
        n201 = Bundle By Name(cluster=w451, "Display settings"=w444) -> (w442:T5)
        n202 = call "Write Display Settings 2 File.vi"("State"=w442) -> ("error out"=w443:errorcluster)  [unwired: 9 in, 1 out]
        n203 = call <vilib>:"Clear Errors.vi"("error in (no error)"=w443) -> ()  [unwired: 5 in, 2 out]
      }
      event Value Change {
        n204 = event-data() -> ("NewVal.Palette Type"=w453:u32, "NewVal.Teiler"=w452:i32)  [unwired: 1 in]
        n205 = call "UserPalette-xRainbows.vi"("Teiler"=w452) -> ("Array"=w454:cluster{u8, u8, u8}[])  [unwired: 1 in]
        n206 = property on="Image" class="ImageControl"("Palette Type"=w453, "User Palette"=w454) -> ()  [unwired: 2 in, 2 out]
      }
      event "Zoom Buttons": Mouse Up {
        n207 = event-data() -> ()  [unwired: 1 in, 2 out]
        n208 = case shown="\"Zoom out\"" "Zoom Buttons" {
          tunnel: [w464 w472 w486] -> w459
          frame "Zoom in", Default {
            n209 = property on="Image" class="ImageControl"() -> (error out=w463:errorcluster, "X Zoom"=w465:i32, "Y Zoom"=w466:i32, "Image Center Position"=w469:cluster{"X":u32, "Y":u32})  [unwired: 2 in, 1 out]
            n210 = Increment(x=w466) -> (x+1=w468:i32)
            n211 = Increment(x=w465) -> (x+1=w467:i32)
            n212 = property on="Image" class="ImageControl"(error in=w463, "X Zoom"=w467, "Y Zoom"=w468, "Image Center Position"=w469) -> (error out=w464:errorcluster)  [unwired: 1 in, 1 out]
          }
          frame "Zoom out" {
            n213 = property on="Image" class="ImageControl"() -> (error out=w470:errorcluster, "X Zoom"=w476:i32, "Y Zoom"=w475:i32, "Image Center Position"=w471:cluster{"X":u32, "Y":u32})  [unwired: 2 in, 1 out]
            n214 = Decrement(x=w476) -> (x-1=w478:i32)
            n215 = Decrement(x=w475) -> (x-1=w477:i32)
            n216 = case shown="0" w478 {
              selector: w478 -> [w482 w485]
              tunnel: w477 -> [w483 w484]
              tunnel: [w481 w485] -> w474
              tunnel: [w480 w484] -> w473
              frame 0 {
                w479 = 2 ("x")
                n217 = Subtract(x=w482, y=w479) -> (x-y=w481:i32)
                n218 = Subtract(x=w483, y=w479) -> (x-y=w480:i32)
              }
              frame 1, Default {
              }
            }
            n219 = property on="Image" class="ImageControl"(error in=w470, "X Zoom"=w474, "Y Zoom"=w473, "Image Center Position"=w471) -> (error out=w472:errorcluster)  [unwired: 1 in, 1 out]
          }
          frame "Zenter" {
            n220 = property on="Centroid" class="Clust (strict)"() -> (error out=w487:errorcluster, "Value"=w488:cluster{"X Centroid":sgl, "Y Centroid":sgl})  [unwired: 2 in, 1 out]
            n221 = property on="Image" class="ImageControl"(error in=w487, "Image Center Position"=w488) -> (error out=w486:errorcluster)  [unwired: 1 in, 1 out]
          }
        }
        n222 = call <vilib>:"Clear Errors.vi"("error in (no error)"=w459) -> ()  [unwired: 5 in, 2 out]
      }
    }
  }
  "Display State Out" <- w4
  "Data Out" <- w7
  "Action" <- w2
